vi "get_scattering_length.vi"(8 "error in (no error)":errorcluster, 11 "GenericTrajectory.lvclass in":refnum<class "TrajectoryDL091126GenericVoxel.lvclass">) -> (0 "error out":errorcluster, 2 "scattering length":dbl[unit], 3 "GenericTrajectory.lvclass out":refnum<class "TrajectoryDL091126GenericVoxel.lvclass">)   [LabVIEW 2010, in "TrajectoryDL091126GenericVoxel.lvclass"]
uses:
  TrajectoryDL091126GenericVoxel.lvclass
  TrajectoryDL091126GenericVoxel.lvclass/TrajectoryDL091126GenericVoxel.ctl
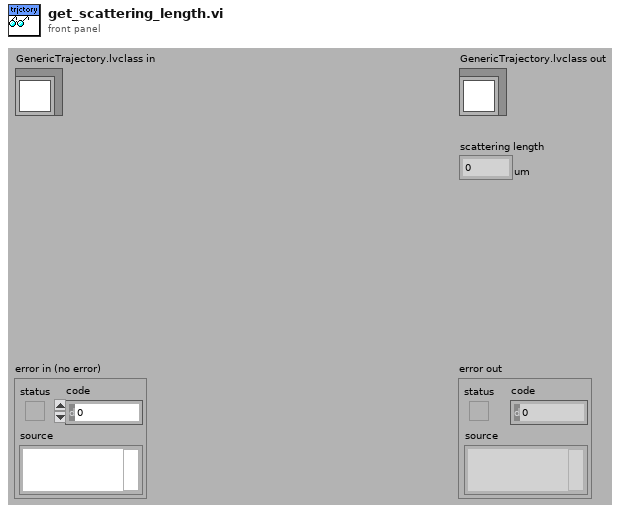
[diagram p1: front panel]
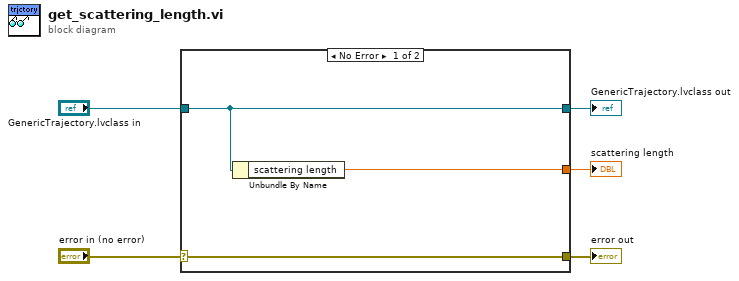
[diagram p0: block diagram]
diagram:
  n1 = case shown="No Error" "error in (no error)" {
    selector: "error in (no error)" -> [w8 w9]
    tunnel: [w8 w9] -> w4
    tunnel: [w7 w10] -> w2
    tunnel: "GenericTrajectory.lvclass in" -> [w7 w10]
    tunnel: [w6 _] -> w1
    frame No Error {
      n2 = Unbundle By Name(w7) -> ("scattering length"=w6:dbl[unit])
    }
    frame Error {
    }
  }
  "error out" <- w4
  "GenericTrajectory.lvclass out" <- w2
  "scattering length" <- w1
